vi "Configure RTD [RTD].vi"(8 "error in (no error)":errorcluster, 9 "resistance (0.0 ohms)":dbl format="%^.2e", 10 "alpha (0.0)":dbl format="%^.2e", 11 "CS++DMM in":refnum<class "CS++DMM.lvclass">) -> (0 "error out":errorcluster, 3 "CS++DMM out":refnum<class "CS++DMM.lvclass">)   [LabVIEW 2013, in "CS++DMM.lvlib" / "CS++DMM.lvclass"]
doc: "This VI configures the alpha and resistance parameters for a resistance temperature device.\n\nThis VI affects the behavior of the instrument only when the IviDmm>Temperature Measurements>Transducer Type [TMP] property is set to IVIDMM_VAL_2_WIRE_RTD or IVIDMM_VAL_4_WIRE_RTD.\n\nNote:\n\n(1) This VI is part of the IviDmmResistanceTemperatureDevice [RTD] extension group.\n\n(2) The driver assumes that you are using a Platinum Resistance Temperature Device."
uses:
  CS++DMM.lvclass
  Core/Classes/CS++ProcessVariables/ProcessVariable/PV.lvclass
  Core/Classes/CS++ProcessVariables/ProcessVariable/PV.lvclass/PV.ctl
  CS++DMM.lvclass/CS++DMM.ctl
  Core/Classes/CS++ProcessVariables/PVConnection/PVConnection.lvclass
  Core/Classes/CS++ProcessVariables/ProcessVariable/Write Data.vi
  Core/Classes/CS++ProcessVariables/ProcessVariable/Write Timestamp.vi
  Core/Classes/CS++ProcessVariables/ProcessVariable/Write Quality.vi
  Core/Classes/CS++ProcessVariables/ProcessVariable/Write status.vi
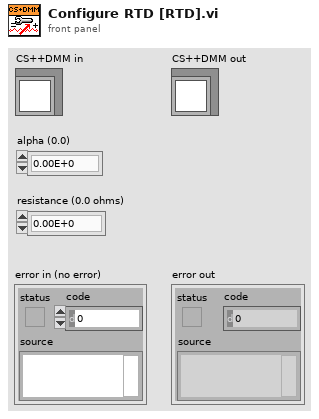
[diagram p1: front panel]
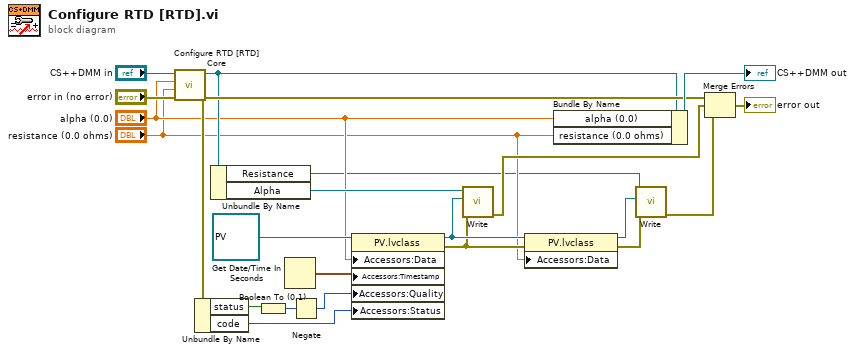
[diagram p0: block diagram]
diagram:
  n1 = call-dynamic "Configure RTD [RTD] Core.vi"("error in (no error)"="error in (no error)", "resistance (0.0 ohms)"="resistance (0.0 ohms)", "alpha (0.0)"="alpha (0.0)", "CS++DMM in"="CS++DMM in") -> ("error out"=w12:errorcluster, "CS++DMM out"=w11:refnum<class "CS++DMM.lvclass">)  [unwired: 6 in]
  n2 = Unbundle By Name(w12) -> ("status"=w18:bool, "code"=w15:i32)
  n3 = Unbundle By Name(w11) -> ("Resistance"=w1:refnum<class "PVConnection.lvclass">, "Alpha"=w13:refnum<class "PVConnection.lvclass">)
  n4 = Boolean To (0,1)(Boolean=w18) -> (0, 1=w17:i16)
  n5 = Get Date/Time In Seconds() -> (seconds since 1Jan1904=w14:timestamp)
  n6 = Negate(x=w17) -> (-x=w16:i16)
  n7 = property class="PV.lvclass"(reference=refnum<class "PV.lvclass"> refnum ("CS++ProcessVariables.lvlib:PV.lvclass"), "Accessors:Data"="alpha (0.0)", "Accessors:Timestamp"=w14, "Accessors:Quality"=w16, "Accessors:Status"=w15) -> (reference out=w4:refnum<class "PV.lvclass">, error out=w3:errorcluster)  [unwired: 1 in]
  n8 = call-dynamic "Write.vi"("error in (no error)"=w3, "PV"=w4, "PVConnection in"=w13) -> ("error out"=w6:errorcluster)  [unwired: 7 in, 1 out]
  n9 = property class="PV.lvclass"(reference=w4, error in=w3, "Accessors:Data"="resistance (0.0 ohms)") -> (reference out=w9:refnum<class "PV.lvclass">, error out=w8:errorcluster)
  n10 = Bundle By Name(cluster=w11, "alpha (0.0)"="alpha (0.0)", "resistance (0.0 ohms)"="resistance (0.0 ohms)") -> (→"CS++DMM out":refnum<class "CS++DMM.lvclass">)
  n11 = call-dynamic "Write.vi"("error in (no error)"=w8, "PV"=w9, "PVConnection in"=w1) -> ("error out"=w5:errorcluster)  [unwired: 7 in, 1 out]
  n12 = Merge Errors(w12, w6, w5) -> (→"error out":errorcluster)
